vi "校准设置页.vi"() -> ()   [LabVIEW 2016, in "斯坦道总氮.lvlib"]
uses:
  <vilib>/Analysis/6fits.llb/Curve Fitting Criteria.ctl
  <vilib>/Analysis/NI_AALPro.lvlib
  <vilib>/ptbypt/NI_PtbyPt.lvlib
panel:
  out "校准状态显示":string caption="校准状态"
  out "刷新时间":string
  out "校准状态":T1(ring)
  out "模型刷新":bool
  in  "校准按钮":T2(radio)
  in  "校准导入":bool
  in  "辅助计算":bool
  in  "曲线模型":T3={"标液浓度1"=0.0, "测量吸光度1"=0.0, "样品1启用"=FALSE, "标液浓度2"=0.0, "测量吸光度2"=0.0, "样品2启用"=FALSE, "标液浓度3"=0.0, "测量吸光度3"=0.0, "样品3启用"=FALSE, "标液浓度4"=0.0, "测量吸光度4"=0.0, "样品4启用"=FALSE, "标液浓度5"=0.0, "测量吸光度5"=0.0, "样品5启用"=FALSE, "模型"=enum."线性", "精度"=4.0, "XY图"=[], "拟合公式"="", "r^2"=0.0, "标样一校准时间"=timestamp(0 s since 1904-01-01), "标样二校准时间"=timestamp(0 s since 1904-01-01), "标样三校准时间"=timestamp(0 s since 1904-01-01), "标样四校准时间"=timestamp(0 s since 1904-01-01), "标样五校准时间"=timestamp(0 s since 1904-01-01), "二次方程"={"c"=0.0, "x"=0.0, "x^2"=0.0}, "标定时间"=timestamp(0 s since 1904-01-01)} {"标定时间" format="%<%m/%d/%y %H:%M:%S>T"; "标样五校准时间" format="%<%m/%d/%y %H:%M:%S>T"; "标样四校准时间" format="%<%m/%d/%y %H:%M:%S>T"; "标样三校准时间" format="%<%m/%d/%y %H:%M:%S>T"; "标样二校准时间" format="%<%m/%d/%y %H:%M:%S>T"; "标样一校准时间" format="%<%m/%d/%y %H:%M:%S>T"; "r^2" format="%.7f"; "测量吸光度5" format="%#.6f"; "测量吸光度4" format="%#.6f"; "测量吸光度3" format="%#.6f"; "测量吸光度2" format="%#.6f"; "测量吸光度1" format="%#.6f"}
  in  "测量模式":T4(ring)
  in  "参数下拉列表":u16(ring)
  in  "量程下拉列表":enum16{"低量程", "高量程"}(ring)
  # "校准时间"
  # "标液浓度"
  # "吸光值"
  # "空白"
  # "标样一"
  # "标样二"
  # "零点"
  # "跨度"
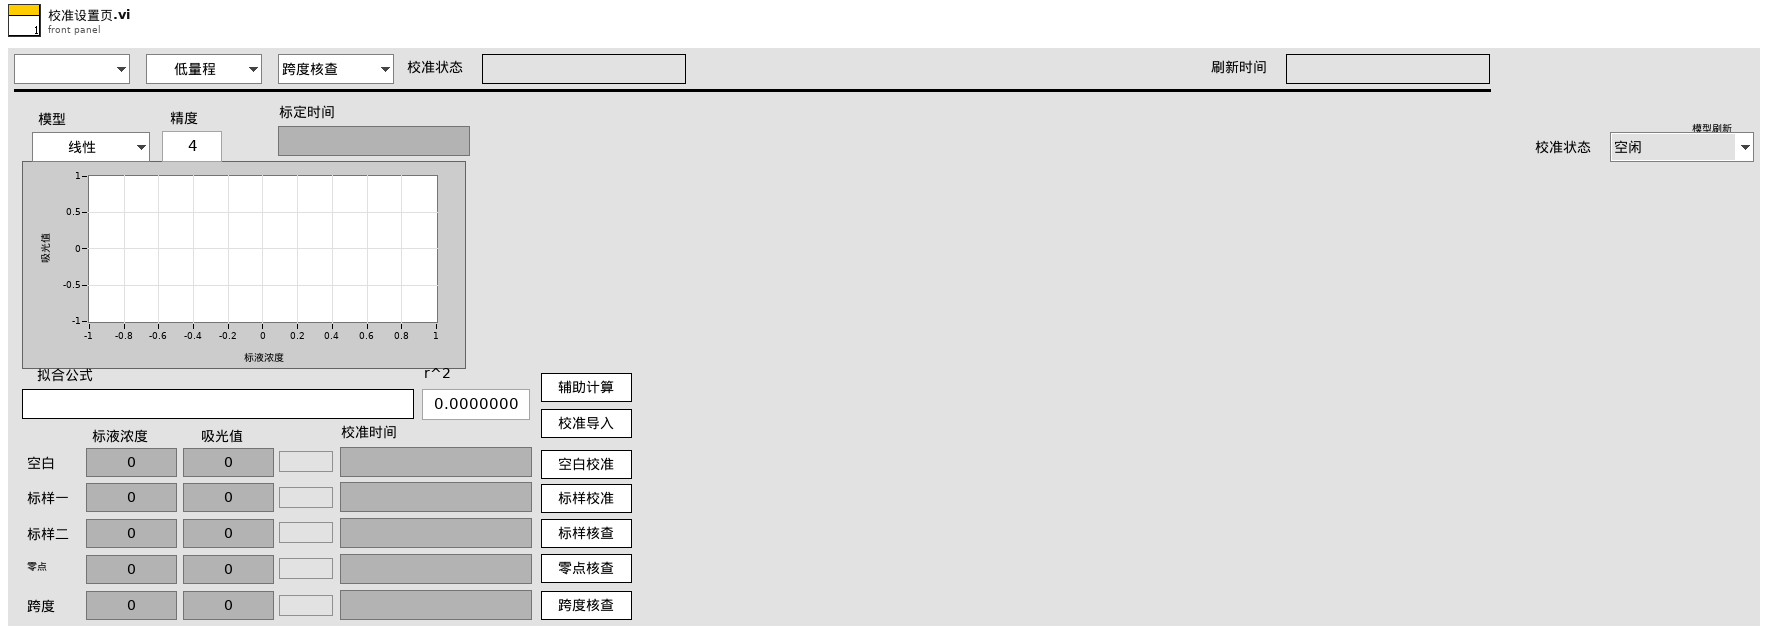
[diagram p1: front panel]
types:
  T1 = enum16{"空闲", "初始化", "校准启动", "校准运行中", "测试结束", "获取校准数据", "填充校准数据", "流程结束"}
  T2 = enum32{"未选择", "空白校准", "标样校准", "标样核查", "零点核查", "跨度核查"}
  T3 = cluster{"标液浓度1":dbl, "测量吸光度1":dbl, "样品1启用":bool, "标液浓度2":dbl, "测量吸光度2":dbl, "样品2启用":bool, "标液浓度3":dbl, "测量吸光度3":dbl, "样品3启用":bool, "标液浓度4":dbl, "测量吸光度4":dbl, "样品4启用":bool, "标液浓度5":dbl, "测量吸光度5":dbl, "样品5启用":bool, "模型":enum32{"线性", "多项式"}, "精度":dbl, "XY图":cluster{"X Values":dbl[], "Y Values":dbl[]}[], "拟合公式":string, "r^2":dbl, "标样一校准时间":timestamp, "标样二校准时间":timestamp, "标样三校准时间":timestamp, "标样四校准时间":timestamp, "标样五校准时间":timestamp, "二次方程":cluster{"c":dbl, "x":dbl, "x^2":dbl}, "标定时间":timestamp}
  T4 = enum16{"跨度核查", "水样测量", "零点核查", "标样核查", "加标回收", "快捷测试", "空白校准", "标样校准"}
  T5 = typedef "LVStringsAndValuesArrayTypeDef_U16.ctl" = cluster{"String":string, "Value":u16}[]
  T6 = enum8{"Enabled", "Disabled", "Disabled and Grayed Out"}
  T7 = cluster{"标液浓度1":dbl, "测量吸光度1":dbl, "样品1启用":bool, "标液浓度2":dbl, "测量吸光度2":dbl, "样品2启用":bool, "标液浓度3":dbl, "测量吸光度3":dbl, "样品3启用":bool, "标液浓度4":dbl, "测量吸光度4":dbl, "样品4启用":bool, "标液浓度5":dbl, "测量吸光度5":dbl, "样品5启用":bool, "模型":enum32{"线性", "多项式"}, "精度":dbl, "XY图":cluster{"X Values":dbl[], "Y Values":dbl[]}[], "拟合公式":string, "r^2":dbl, "标样一校准时间":timestamp, "标样二校准时间":timestamp, "标样三校准时间":timestamp, "标样四校准时间":timestamp, "标样五校准时间":timestamp, "二次方程":cluster{"c":dbl, "x":dbl, "x^2":dbl}, "标定时间":timestamp}[][]
  T8 = typedef "NI_AALPro.lvlib/Curve Fitting Criteria.ctl" = u16
  T9 = cluster{"标液浓度1":dbl, "测量吸光度1":dbl, "样品1启用":bool, "标液浓度2":dbl, "测量吸光度2":dbl, "样品2启用":bool, "标液浓度3":dbl, "测量吸光度3":dbl, "样品3启用":bool, "标液浓度4":dbl, "测量吸光度4":dbl, "样品4启用":bool, "标液浓度5":dbl, "测量吸光度5":dbl, "样品5启用":bool, "模型":enum32{"线性", "多项式"}, "精度":dbl, "XY图":cluster{"X Values":dbl[], "Y Values":dbl[]}[], "拟合公式":string, "r^2":dbl, "标样一校准时间":timestamp, "标样二校准时间":timestamp, "标样三校准时间":timestamp, "标样四校准时间":timestamp, "标样五校准时间":timestamp, "二次方程":cluster{"c":dbl, "x":dbl, "x^2":dbl}, "标定时间":timestamp}[]
  T10 = enum32{"Bad", "Idle", "Run top level", "Running"}
  T11 = cluster{"时间":timestamp, "标液值":dbl, "检测值":dbl, "吸光值":dbl}
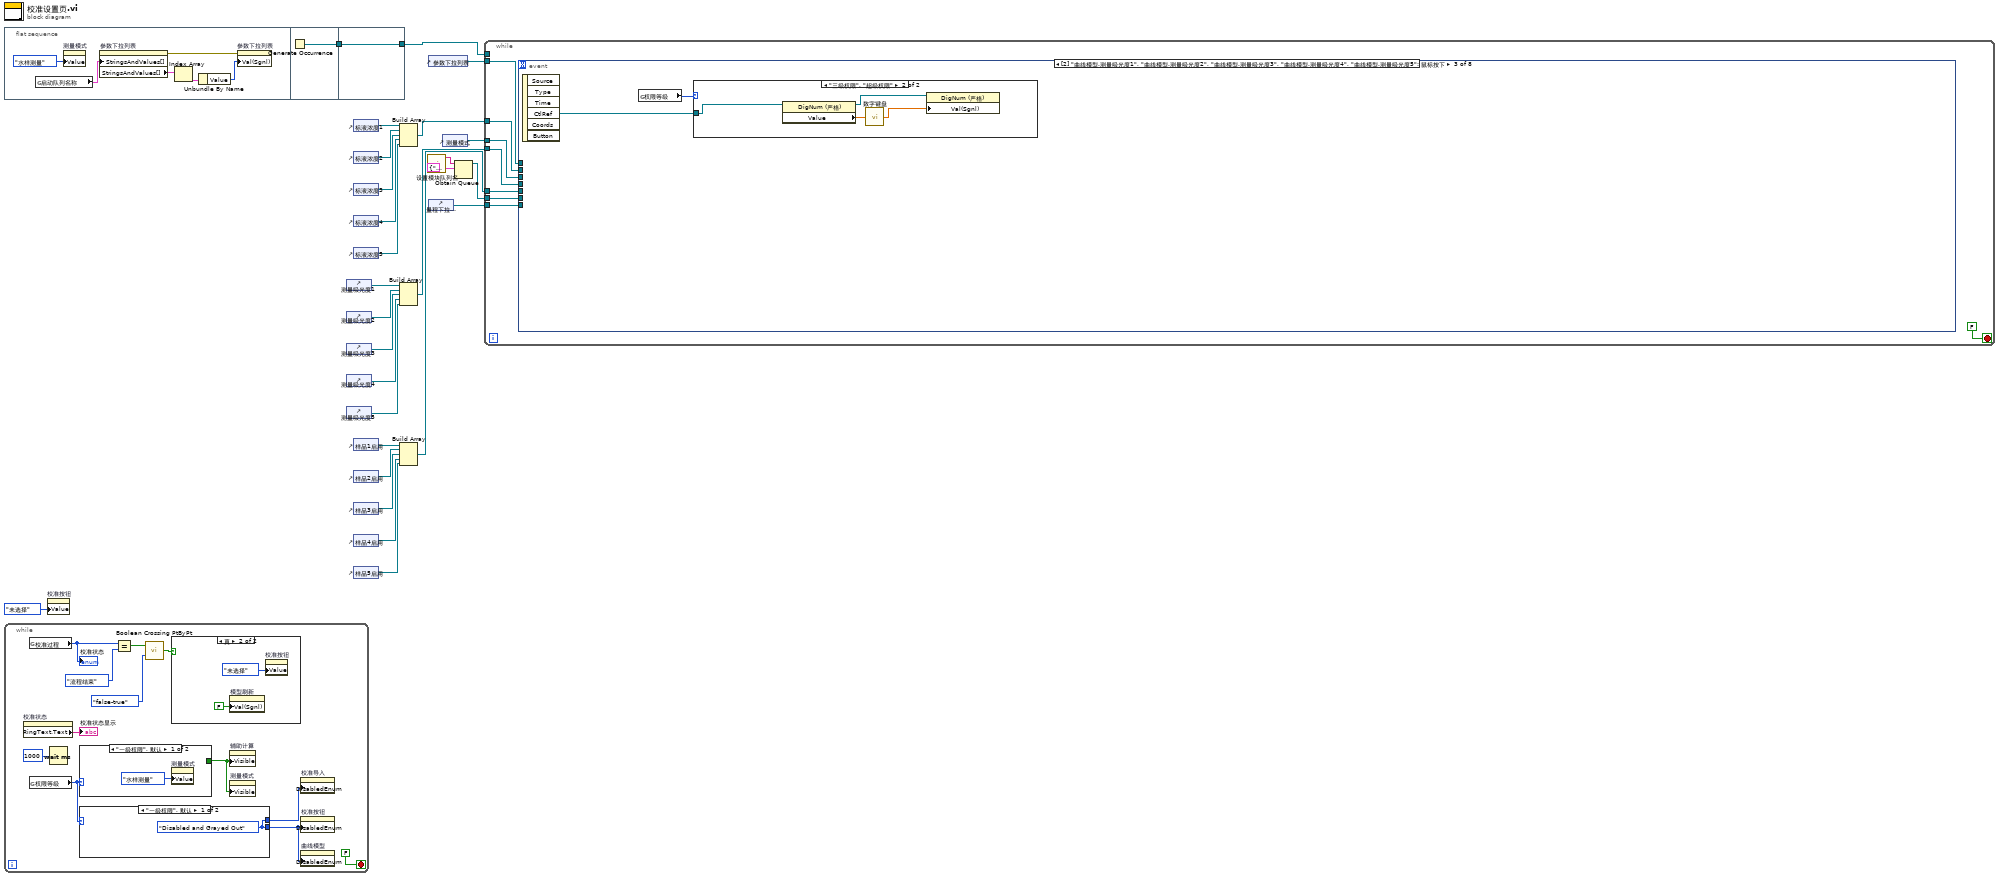
[diagram p0: block diagram]
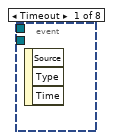
[diagram p2: hidden frame]
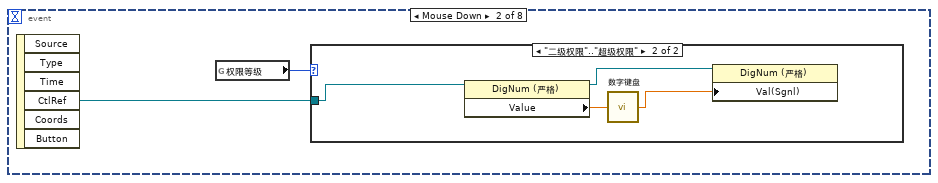
[diagram p3: hidden frame]
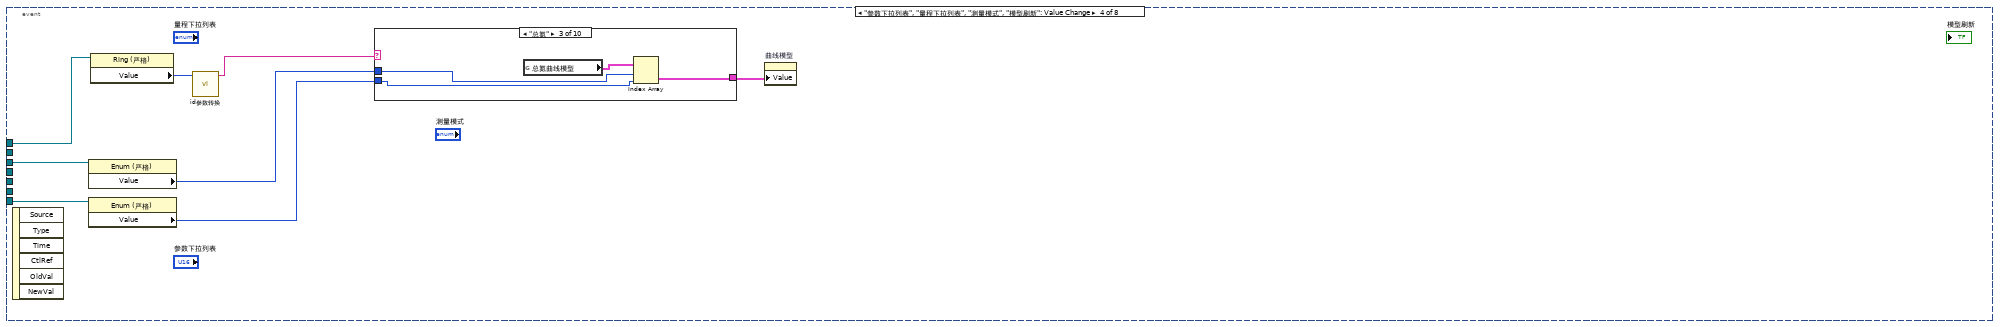
[diagram p6: hidden frame]
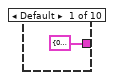
[diagram p7: hidden frame]
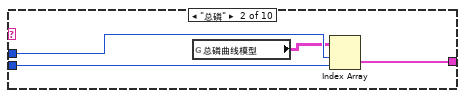
[diagram p8: hidden frame]
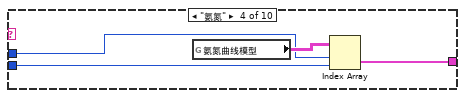
[diagram p9: hidden frame]
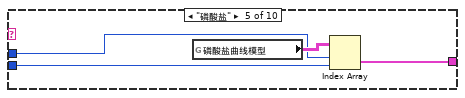
[diagram p10: hidden frame]
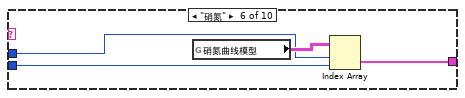
[diagram p11: hidden frame]
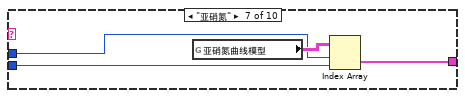
[diagram p12: hidden frame]
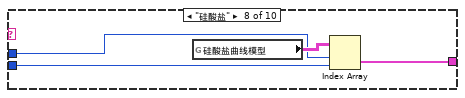
[diagram p13: hidden frame]
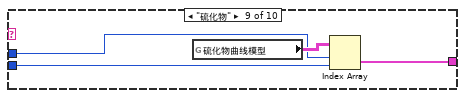
[diagram p14: hidden frame]
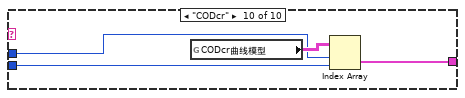
[diagram p15: hidden frame]
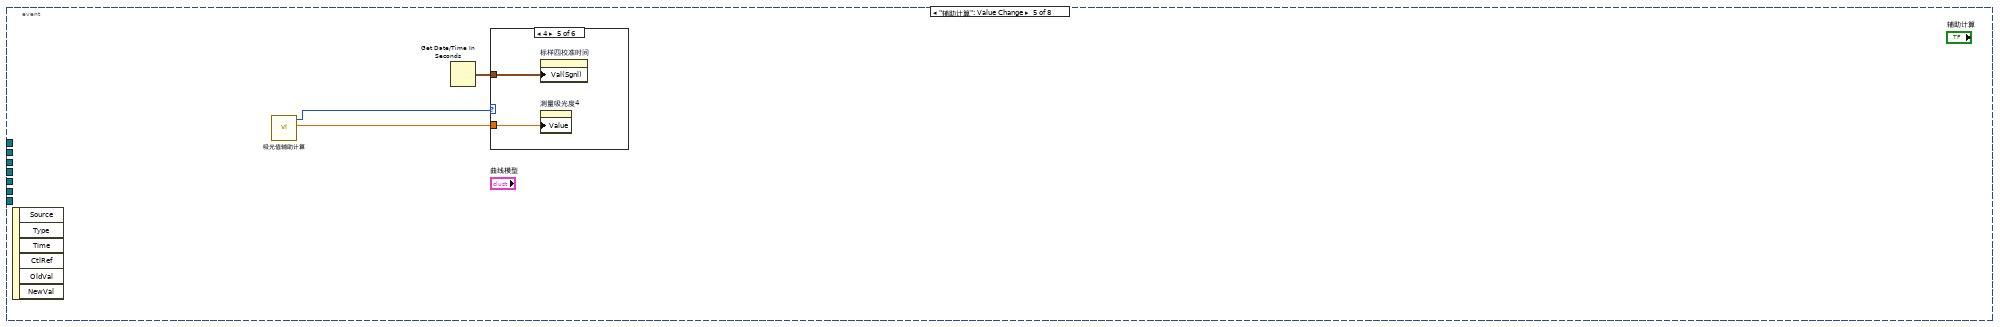
[diagram p16: hidden frame]
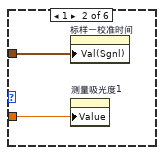
[diagram p18: hidden frame]
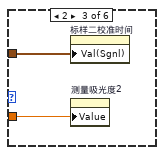
[diagram p19: hidden frame]
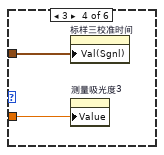
[diagram p20: hidden frame]
diagram:
  n1 = flat-sequence {
    tunnel: [w34] -> w27
    tunnel: [w35] -> w26
    tunnel: w27 -> [w35]
    frame #0 {
      n2 = global read "总磷总氮断电保存全局变量.vi" "启动队列名称"() -> (w29:cluster{"String":string, "Value":u16}[])
      n3 = property on="测量模式" class="Enum (严格)"("Value"=T4."水样测量" ("测量模式")) -> ()  [unwired: 2 in, 2 out]
      n4 = property on="参数下拉列表" class="Ring (严格)"("StringsAndValues[]"=w29) -> (error out=w32:errorcluster, "StringsAndValues[]"=w30:T5)  [unwired: 2 in, 1 out]
      n5 = Index Array(array=w30) -> (element=w31:cluster{"String":string, "Value":u16})  [unwired: 1 in]
      n6 = Unbundle By Name(w31) -> ("Value"=w33:u16)
      n7 = property on="参数下拉列表" class="Ring (严格)"(error in=w32, "Val(Sgnl)"=w33) -> ()  [unwired: 1 in, 2 out]
    }
    frame #1 {
      n8 = Generate Occurrence() -> (w34:refnum<k4>)
    }
    frame #2 {
    }
  }
  n9 = while {
    stop <- FALSE stop-if-true
    n10 = property on="校准状态" class="Enum (严格)"() -> ("RingText.Text"=→"校准状态显示":string)  [unwired: 2 in, 2 out]
    n11 = global read "VAR总磷总氮全局变量.vi" "校准过程"() -> (w38:T1)
    "校准状态" <- w38
    n12 = global read "VAR总磷总氮全局变量.vi" "权限等级"() -> (w44:enum16{"一级权限", "二级权限", "三级权限", "超级权限"})
    n13 = Wait (ms)(milliseconds to wait=u32 1000 ("等待时间（毫秒）")) -> ()  [unwired: 1 out]
    n14 = case shown="\"一级权限\", 默认" w44 {
      tunnel: [_ TRUE ("可见")] -> w43
      frame "一级权限", Default {
        n15 = property on="测量模式" class="Enum (严格)"("Value"=T4."水样测量" ("测量模式")) -> ()  [unwired: 2 in, 2 out]
      }
      frame "三级权限", "超级权限" {
      }
    }
    n16 = case shown="\"一级权限\", 默认" w44 {
      tunnel: [w52 w53] -> w42
      tunnel: [w52 w53] -> w45
      frame "一级权限", Default {
        w52 = T6."Disabled and Grayed Out" ("禁用")
      }
      frame "二级权限".."超级权限" {
        w53 = T6."Enabled" ("禁用")
      }
    }
    n17 = Equal?(x=w38, y=T1."流程结束" ("校准过程")) -> (x = y?=w41:bool)
    n18 = call <vilib>:"Boolean Crossing PtByPt.vi"("direction"=enum16{"either", "false-true", "true-false"}."false-true", "input"=w41) -> ("crossing"=w39:bool)  [unwired: 1 in]
    n19 = case shown="真" w39 {
      frame False {
      }
      frame True {
        n20 = property on="模型刷新" class="Bool (严格)"("Val(Sgnl)"=FALSE ("值(信号)")) -> ()  [unwired: 2 in, 2 out]
        n21 = property on="校准按钮" class="RadioBtnsControl (严格)"("Value"=T2."未选择" ("校准按钮")) -> ()  [unwired: 2 in, 2 out]
      }
    }
    n22 = property on="辅助计算" class="Bool"("Visible"=w43) -> ()  [unwired: 2 in, 2 out]
    n23 = property on="测量模式" class="Enum (严格)"("Visible"=w43) -> ()  [unwired: 2 in, 2 out]
    n24 = property on="校准导入" class="Bool"("DisabledEnum"=w45) -> ()  [unwired: 2 in, 2 out]
    n25 = property on="校准按钮" class="RadioBtnsControl (严格)"("DisabledEnum"=w42) -> ()  [unwired: 2 in, 2 out]
    n26 = property on="曲线模型" class="Clust (严格)"("DisabledEnum"=w42) -> ()  [unwired: 2 in, 2 out]
  }
  n27 = property on="校准按钮" class="RadioBtnsControl (严格)"("Value"=T2."未选择" ("校准按钮")) -> ()  [unwired: 2 in, 2 out]
  n28 = control-ref of="测量吸光度1"() -> (w15:refnum<vi>)
  n29 = control-ref of="测量吸光度2"() -> (w16:refnum<vi>)
  n30 = control-ref of="测量吸光度3"() -> (w17:refnum<vi>)
  n31 = control-ref of="测量吸光度4"() -> (w18:refnum<vi>)
  n32 = control-ref of="测量吸光度5"() -> (w19:refnum<vi>)
  n33 = control-ref of="标液浓度1"() -> (w13:refnum<vi>)
  n34 = control-ref of="标液浓度2"() -> (w12:refnum<vi>)
  n35 = control-ref of="标液浓度3"() -> (w11:refnum<vi>)
  n36 = control-ref of="标液浓度4"() -> (w10:refnum<vi>)
  n37 = control-ref of="标液浓度5"() -> (w9:refnum<vi>)
  n38 = control-ref of="样品1启用"() -> (w25:refnum<vi>)
  n39 = control-ref of="样品2启用"() -> (w24:refnum<vi>)
  n40 = control-ref of="样品3启用"() -> (w23:refnum<vi>)
  n41 = control-ref of="样品4启用"() -> (w22:refnum<vi>)
  n42 = control-ref of="样品5启用"() -> (w21:refnum<vi>)
  n43 = Build Array(w13, w12, w11, w10, w9) -> (w8:refnum<vi>[])
  n44 = Build Array(w15, w16, w17, w18, w19) -> (w14:refnum<vi>[])
  n45 = Build Array(w25, w24, w23, w22, w21) -> (w20:refnum<vi>[])
  n46 = call "设置模块队列名.vi"() -> ("Msg"=w6:string)  [unwired: 5 in]
  n47 = control-ref of="参数下拉列表"() -> (w3:refnum<vi>)
  n48 = control-ref of="量程下拉列表"() -> (w1:refnum<vi>)
  n49 = control-ref of="测量模式"() -> (w2:refnum<vi>)
  n50 = Obtain Queue(name (unnamed)=w6, element data type=cluster{"命令":string, "data":variant} {"命令"="", "data"=variant}) -> (queue out=w5:refnum<queue>)  [unwired: 3 in, 2 out]
  n51 = while {
    tunnel: w26 -> [_]
    tunnel: w3 -> [w60]
    tunnel: w20 -> [w59]
    tunnel: w14 -> [w58]
    tunnel: w8 -> [w57]
    tunnel: w2 -> [w56]
    tunnel: w1 -> [w55]
    tunnel: w5 -> [w54]
    stop <- FALSE stop-if-true
    n52 = event shown="[2] \"曲线模型.测量吸光度1\", \"曲线模型.测量吸光度2\", \"曲线模型.测量吸光度3\", \"曲线模型.测量吸光度4\", \"曲线模型.测量吸光度5\": 鼠标按下" {
      selector: _ -> [_ _ _ _ _ _ _ _]
      dyn-events: _ -> [_ _ _ _ _ _ _ _]
      timeout: _ -> [_ _ _ _ _ _ _ _]
      tunnel: w60 -> [_ _ _ w80 _ w144 w190 w272]
      tunnel: w59 -> [_ _ _ _ _ _ w194 _]
      tunnel: w58 -> [_ _ _ _ _ _ w193 _]
      tunnel: w57 -> [_ _ _ _ _ _ w192 _]
      tunnel: w56 -> [_ _ _ w78 _ w142 w188 w267]
      tunnel: w55 -> [_ _ _ w77 _ w140 w186 w271]
      tunnel: w54 -> [_ _ _ _ _ _ _ w273]
      event Timeout {
        n53 = event-data() -> ()  [unwired: 1 in, 3 out]
      }
      event "曲线模型.标液浓度1", "曲线模型.标液浓度2", "曲线模型.标液浓度3", "曲线模型.标液浓度4", "曲线模型.标液浓度5", "曲线模型.精度": Mouse Down {
        n54 = event-data() -> ("CtlRef"=w63:refnum<vi>)  [unwired: 1 in, 5 out]
        n55 = global read "VAR总磷总氮全局变量.vi" "权限等级"() -> (w62:enum16{"一级权限", "二级权限", "三级权限", "超级权限"})
        n56 = case shown="\"二级权限\"..\"超级权限\"" w62 {
          tunnel: w63 -> [_ w67]
          frame "一级权限", Default {
          }
          frame "二级权限".."超级权限" {
            n57 = property class="DigNum (严格)"(reference=w67) -> (reference out=w65:refnum<vi>, "Value"=w66:dbl)  [unwired: 1 in, 1 out]
            n58 = call "数字键盘.vi"("OldNumber"=w66) -> ("NewNumber"=w64:dbl)
            n59 = property class="DigNum (严格)"(reference=w65, "Val(Sgnl)"=w64) -> ()  [unwired: 1 in, 2 out]
          }
        }
      }
      event "曲线模型.测量吸光度1", "曲线模型.测量吸光度2", "曲线模型.测量吸光度3", "曲线模型.测量吸光度4", "曲线模型.测量吸光度5": Mouse Down {
        n60 = event-data() -> ("CtlRef"=w69:refnum<vi>)  [unwired: 1 in, 5 out]
        n61 = global read "VAR总磷总氮全局变量.vi" "权限等级"() -> (w68:enum16{"一级权限", "二级权限", "三级权限", "超级权限"})
        n62 = case shown="\"三级权限\", \"超级权限\"" w68 {
          tunnel: w69 -> [_ w73]
          frame "一级权限", Default {
          }
          frame "三级权限", "超级权限" {
            n63 = property class="DigNum (严格)"(reference=w73) -> (reference out=w71:refnum<vi>, "Value"=w72:dbl)  [unwired: 1 in, 1 out]
            n64 = call "数字键盘.vi"("OldNumber"=w72) -> ("NewNumber"=w70:dbl)
            n65 = property class="DigNum (严格)"(reference=w71, "Val(Sgnl)"=w70) -> ()  [unwired: 1 in, 2 out]
          }
        }
      }
      event "参数下拉列表", "量程下拉列表", "测量模式", "模型刷新": Value Change {
        n66 = event-data() -> ()  [unwired: 1 in, 6 out]
        n67 = property class="Enum (严格)"(reference=w78) -> ("Value"=w75:T4)  [unwired: 1 in, 2 out]
        n68 = property class="Enum (严格)"(reference=w77) -> ("Value"=w74:enum16{"低量程", "高量程"})  [unwired: 1 in, 2 out]
        n69 = property class="Ring (严格)"(reference=w80) -> ("Value"=w81:u16)  [unwired: 1 in, 2 out]
        n70 = call "id参数转换.vi"("id"=w81) -> ("table输出"=w79:string)  [unwired: 9 in, 1 out]
        n71 = case shown="\"总氮\"" w79 {
          tunnel: w74 -> [_ w85 w90 w92 w96 w100 w104 w108 w112 w116]
          tunnel: w75 -> [_ w86 w89 w93 w97 w101 w105 w109 w113 w117]
          tunnel: [T3 {"标液浓度1"=0.0, "测量吸光度1"=0.0, "样品1启用"=FALSE, "标液浓度2"=0.0, "测量吸光度2"=0.0, "样品2启用"=FALSE, "标液浓度3"=0.0, "测量吸光度3"=0.0, "样品3启用"=FALSE, "标液浓度4"=0.0, "测量吸光度4"=0.0, "样品4启用"=FALSE, "标液浓度5"=0.0, "测量吸光度5"=0.0, "样品5启用"=FALSE, "模型"=enum."线性", "精度"=0.0, "XY图"=[], "拟合公式"="", "r^2"=0.0, "标样一校准时间"=timestamp(0 s since 1904-01-01), "标样二校准时间"=timestamp(0 s since 1904-01-01), "标样三校准时间"=timestamp(0 s since 1904-01-01), "标样四校准时间"=timestamp(0 s since 1904-01-01), "标样五校准时间"=timestamp(0 s since 1904-01-01), "二次方程"={"c"=0.0, "x"=0.0, "x^2"=0.0}, "标定时间"=timestamp(0 s since 1904-01-01)} ("总磷曲线模型") w83 w87 w91 w95 w99 w103 w107 w111 w115] -> w76
          frame Default {
          }
          frame "总磷" {
            n72 = global read "校准数据全局变量.vi" "总磷曲线模型"() -> (w84:T7)
            n73 = Index Array(array=w84, index (row)=w86, index (col)=w85) -> (element=w83:T3)
          }
          frame "总氮" {
            n74 = global read "校准数据全局变量.vi" "总氮曲线模型"() -> (w88:T7)
            n75 = Index Array(array=w88, index (row)=w89, index (col)=w90) -> (element=w87:T3)
          }
          frame "氨氮" {
            n76 = global read "校准数据全局变量.vi" "氨氮曲线模型"() -> (w94:T7)
            n77 = Index Array(array=w94, index (row)=w93, index (col)=w92) -> (element=w91:T3)
          }
          frame "磷酸盐" {
            n78 = global read "校准数据全局变量.vi" "磷酸盐曲线模型"() -> (w98:T7)
            n79 = Index Array(array=w98, index (row)=w97, index (col)=w96) -> (element=w95:T3)
          }
          frame "硝氮" {
            n80 = global read "校准数据全局变量.vi" "硝氮曲线模型"() -> (w102:T7)
            n81 = Index Array(array=w102, index (row)=w101, index (col)=w100) -> (element=w99:T3)
          }
          frame "亚硝氮" {
            n82 = global read "校准数据全局变量.vi" "亚硝氮曲线模型"() -> (w106:T7)
            n83 = Index Array(array=w106, index (row)=w105, index (col)=w104) -> (element=w103:T3)
          }
          frame "硅酸盐" {
            n84 = global read "校准数据全局变量.vi" "硅酸盐曲线模型"() -> (w110:T7)
            n85 = Index Array(array=w110, index (row)=w109, index (col)=w108) -> (element=w107:T3)
          }
          frame "硫化物" {
            n86 = global read "校准数据全局变量.vi" "硫化物曲线模型"() -> (w114:T7)
            n87 = Index Array(array=w114, index (row)=w113, index (col)=w112) -> (element=w111:T3)
          }
          frame "CODcr" {
            n88 = global read "校准数据全局变量.vi" "CODcr曲线模型"() -> (w118:T7)
            n89 = Index Array(array=w118, index (row)=w117, index (col)=w116) -> (element=w115:T3)
          }
        }
        n90 = property on="曲线模型" class="Clust (严格)"("Value"=w76) -> ()  [unwired: 2 in, 2 out]
      }
      event "辅助计算": Value Change {
        n91 = event-data() -> ()  [unwired: 1 in, 6 out]
        n92 = call "吸光值辅助计算.vi"() -> ("X"=w120:dbl, "吸光值导出"=w121:u16)  [unwired: 10 in]
        n93 = Get Date/Time In Seconds() -> (seconds since 1Jan1904=w119:timestamp)
        n94 = case shown="4" w121 {
          tunnel: w120 -> [_ w123 w125 w127 w129 w131]
          tunnel: w119 -> [_ w122 w124 w126 w128 w130]
          frame 0, Default {
          }
          frame 1 {
            n95 = property on="标样一校准时间" class="AbsTime (严格)"("Val(Sgnl)"=w122) -> ()  [unwired: 2 in, 2 out]
            n96 = property on="测量吸光度1" class="DigNum (严格)"("Value"=w123) -> ()  [unwired: 2 in, 2 out]
          }
          frame 2 {
            n97 = property on="标样二校准时间" class="AbsTime (严格)"("Val(Sgnl)"=w124) -> ()  [unwired: 2 in, 2 out]
            n98 = property on="测量吸光度2" class="DigNum (严格)"("Value"=w125) -> ()  [unwired: 2 in, 2 out]
          }
          frame 3 {
            n99 = property on="标样三校准时间" class="AbsTime (严格)"("Val(Sgnl)"=w126) -> ()  [unwired: 2 in, 2 out]
            n100 = property on="测量吸光度3" class="DigNum (严格)"("Value"=w127) -> ()  [unwired: 2 in, 2 out]
          }
          frame 4 {
            n101 = property on="标样四校准时间" class="AbsTime (严格)"("Val(Sgnl)"=w128) -> ()  [unwired: 2 in, 2 out]
            n102 = property on="测量吸光度4" class="DigNum (严格)"("Value"=w129) -> ()  [unwired: 2 in, 2 out]
          }
          frame 5 {
            n103 = property on="标样五校准时间" class="AbsTime (严格)"("Val(Sgnl)"=w130) -> ()  [unwired: 2 in, 2 out]
            n104 = property on="测量吸光度5" class="DigNum (严格)"("Value"=w131) -> ()  [unwired: 2 in, 2 out]
          }
        }
      }
      event "校准导入": Value Change {
        n105 = event-data() -> ()  [unwired: 1 in, 6 out]
        n106 = property class="Enum (严格)"(reference=w142) -> ("Value"=w141:T4)  [unwired: 1 in, 2 out]
        n107 = property class="Enum (严格)"(reference=w140) -> ("Value"=w139:enum16{"低量程", "高量程"})  [unwired: 1 in, 2 out]
        n108 = property class="Ring (严格)"(reference=w144) -> ("Value"=w143:u16)  [unwired: 1 in, 2 out]
        n109 = property on="二次方程" class="Clust (严格)"() -> ("Value"=w133:cluster{"c":dbl, "x":dbl, "x^2":dbl})  [unwired: 2 in, 2 out]
        n110 = Unbundle By Name(w133) -> ("x^2"=w135:dbl, "x"=w136:dbl, "c"=w137:dbl)
        n111 = Bundle By Name(cluster=cluster{"X^2":dbl, "X":dbl, "b":dbl} {"X^2"=0.0, "X"=0.0, "b"=0.0} ("公式"), "X^2"=w135, "X"=w136, "b"=w137) -> (w132:cluster{"X^2":dbl, "X":dbl, "b":dbl})
        n112 = global read "VAR总磷总氮全局变量.vi" "权限等级"() -> (w138:enum16{"一级权限", "二级权限", "三级权限", "超级权限"})
        n113 = case shown="\"三级权限\", \"超级权限\"" w138 {
          tunnel: w143 -> [w153 w184]
          tunnel: w141 -> [w152 w183]
          tunnel: w139 -> [w151 w182]
          tunnel: w132 -> [w145 _]
          frame "一级权限", Default {
            n114 = Cluster To Array(cluster=w145) -> (array=w150:dbl[])
            n115 = Add Array Elements(numeric array=w150) -> (sum=w149:dbl)
            n116 = Equal To 0?(x=w149) -> (x = 0?=w147:bool)
            n117 = Not A Number/Path/Refnum?(number/path/refnum=w149) -> (NaN/Path/Refnum?=w148:bool)
            n118 = Or(x=w147, y=w148) -> (x .or. y?=w146:bool)
            n119 = case shown="假" w146 {
              tunnel: w153 -> [w159 _]
              tunnel: w152 -> [w158 _]
              tunnel: w151 -> [w157 _]
              tunnel: w145 -> [w154 _]
              frame False {
                n120 = Two Button Dialog(message="请再一次确认是否导入" ("消息")) -> (T button?=w155:bool)  [unwired: 2 in]
                n121 = case shown="真" w155 {
                  tunnel: w159 -> [_ w161]
                  tunnel: w158 -> [_ w167]
                  tunnel: w157 -> [_ w160]
                  tunnel: w154 -> [_ w162]
                  frame False {
                  }
                  frame True {
                    n122 = for {
                      N: 8 -> [_]
                      tunnel: w161 -> [w173]
                      tunnel: w167 -> [_]
                      tunnel: w160 -> [w172]
                      shift-right: [w171] -> w165
                      shift-left: errorcluster {"status"=FALSE, "code"=0, "source"=""} ("error out") -> [w168]
                      tunnel: w162 -> [w169]
                      i -> [w170]
                      n123 = call "总磷总氮公式写入.vi"("公式"=w169, "error in (no error)"=w168, "量程"=w172, "测量模式"=w170, "测量参数"=w173) -> ("error out"=w171:errorcluster)  [unwired: 6 in]
                    }
                    n124 = case shown="无错误" w165 {
                      tunnel: ["写入成功" "写入失败"] -> w166
                      tunnel: w161 -> [w177 _]
                      tunnel: w160 -> [w176 _]
                      frame No Error {
                        n125 = Get Date/Time In Seconds() -> (seconds since 1Jan1904=w178:timestamp)
                        n126 = property on="标定时间" class="AbsTime (严格)"("Val(Sgnl)"=w178) -> (error out=w174:errorcluster)  [unwired: 2 in, 1 out]
                        n127 = property on="曲线模型" class="Clust (严格)"(error in=w174) -> ("Value"=w175:T3)  [unwired: 1 in, 2 out]
                        n128 = call "校准记录.vi"("曲线模型"=w175, "量程"=w176, "校准参数"=w177) -> ()  [unwired: 8 in, 1 out]
                      }
                      frame Error {
                      }
                    }
                    n129 = One Button Dialog(message=w166) -> ()  [unwired: 1 in, 1 out]
                  }
                }
              }
              frame True {
                n130 = One Button Dialog(message="校准数据异常，请重新校准！" ("消息")) -> ()  [unwired: 1 in, 1 out]
              }
            }
          }
          frame "三级权限", "超级权限" {
            n131 = call "公式复合写入.vi"("量程下拉列表"=w182, "测量模式"=w183, "参数下拉列表"=w184) -> ()  [unwired: 9 in]
          }
        }
      }
      event "曲线模型": Value Change {
        n132 = event-data() -> ()  [unwired: 1 in, 6 out]
        n133 = flat-sequence {
          tunnel: w194 -> [w214]
          tunnel: w193 -> [w212]
          tunnel: w192 -> [w210]
          tunnel: [w197] -> w191
          tunnel: w190 -> [w197]
          tunnel: [w196] -> w189
          tunnel: w188 -> [w196]
          tunnel: [w195] -> w187
          tunnel: w186 -> [w195]
          tunnel: w191 -> [w230]
          tunnel: w189 -> [w227]
          tunnel: w187 -> [w226]
          frame #0 {
            w206 = T8 0 items=["最小二乘", "最小绝对残差", "Bisquare"] ("method")
            n134 = for {
              tunnel: w214 -> [w220] mode=indexing
              tunnel: [w219] -> w213 mode=indexing
              tunnel: w212 -> [w218] mode=indexing
              tunnel: [w217] -> w211 mode=indexing
              tunnel: w210 -> [w216] mode=indexing
              tunnel: [w215] -> w209 mode=indexing
              n135 = property class="DigNum (严格)"(reference=w216) -> ("Value"=w215:dbl)  [unwired: 1 in, 2 out]
              n136 = property class="DigNum (严格)"(reference=w218) -> ("Value"=w217:dbl)  [unwired: 1 in, 2 out]
              n137 = property class="Bool (严格)"(reference=w220) -> ("Value"=w219:bool)  [unwired: 1 in, 2 out]
            }
            n138 = property on="模型" class="Enum (严格)"() -> ("Value"=w208:enum32{"线性", "多项式"})  [unwired: 2 in, 2 out]
            n139 = property on="精度" class="DigNum (严格)"() -> ("Value"=w207:dbl)  [unwired: 2 in, 2 out]
            n140 = call "线性公式.vi"("精度"=w207, "模型"=w208, "method"=w206, "启用"=w213, "监测浓度"=w211, "标液浓度"=w209) -> ("Polynomial Coefficients 2"=w202:dbl[], "XY图"=w203:cluster{"X Values":dbl[], "Y Values":dbl[]}[], "r^2"=w204:dbl, "拟合方程"=w205:string)  [unwired: 2 in]
            n141 = property on="拟合公式" class="Str"("Value"=w205) -> ()  [unwired: 2 in, 2 out]
            n142 = property on="r^2" class="DigNum (严格)"("Value"=w204) -> ()  [unwired: 2 in, 2 out]
            n143 = property on="XY图" class="XYGraph (严格)"("Value"=w203) -> ()  [unwired: 2 in, 2 out]
            n144 = Index Array(array=w202) -> (element #1=w201:dbl, element #2=w200:dbl, element #3=w199:dbl)  [unwired: 3 in]
            n145 = Bundle("slope"=w201, "slope"=w200, "slope"=w199) -> (w198:cluster{"slope":dbl, "slope":dbl, "slope":dbl})  [unwired: 1 in]
            n146 = property on="二次方程" class="Clust (严格)"("Value"=w198) -> ()  [unwired: 2 in, 2 out]
          }
          frame #1 {
            n147 = property class="Enum (严格)"(reference=w227) -> ("Value"=w224:T4)  [unwired: 1 in, 2 out]
            n148 = property class="Enum (严格)"(reference=w226) -> ("Value"=w225:enum16{"低量程", "高量程"})  [unwired: 1 in, 2 out]
            n149 = property class="Ring (严格)"(reference=w230) -> ("Value"=w229:u16)  [unwired: 1 in, 2 out]
            n150 = property on="曲线模型" class="Clust (严格)"() -> ("Value"=w222:T3)  [unwired: 2 in, 2 out]
            n151 = call "id参数转换.vi"("id"=w229) -> ("table输出"=w228:string)  [unwired: 9 in, 1 out]
            n152 = Initialize Array(w222, 10 ("维数大小")) -> (w221:T9)
            n153 = case shown="\"总磷\"" w228 {
              tunnel: w221 -> [_ w231 w238 w240 w243 w247 w251 w255 w259 w264]
              tunnel: w225 -> [_ w234 w237 w241 w244 w248 w252 w256 w260 w265]
              tunnel: w224 -> [_ _ _ _ _ _ _ _ _ _]
              frame Default {
              }
              frame "总磷" {
                n154 = global read "校准数据全局变量.vi" "总磷曲线模型"() -> (w232:T7)
                n155 = Replace Array Subset(array=w232, new element=w231, index (col)=w234) -> (w233:T7)  [unwired: 1 in]
                n156 = global write "校准数据全局变量.vi" "总磷曲线模型"(w233) -> ()
              }
              frame "总氮" {
                n157 = global read "校准数据全局变量.vi" "总氮曲线模型"() -> (w236:T7)
                n158 = Replace Array Subset(array=w236, new element=w238, index (col)=w237) -> (w235:T7)  [unwired: 1 in]
                n159 = global write "校准数据全局变量.vi" "总氮曲线模型"(w235) -> ()
              }
              frame "氨氮" {
                n160 = global read "校准数据全局变量.vi" "氨氮曲线模型"() -> (w242:T7)
                n161 = Replace Array Subset(array=w242, new element=w240, index (col)=w241) -> (w239:T7)  [unwired: 1 in]
                n162 = global write "校准数据全局变量.vi" "氨氮曲线模型"(w239) -> ()
              }
              frame "磷酸盐" {
                n163 = global read "校准数据全局变量.vi" "磷酸盐曲线模型"() -> (w246:T7)
                n164 = Replace Array Subset(array=w246, new element=w243, index (col)=w244) -> (w245:T7)  [unwired: 1 in]
                n165 = global write "校准数据全局变量.vi" "磷酸盐曲线模型"(w245) -> ()
              }
              frame "硝氮" {
                n166 = global read "校准数据全局变量.vi" "硝氮曲线模型"() -> (w250:T7)
                n167 = Replace Array Subset(array=w250, new element=w247, index (col)=w248) -> (w249:T7)  [unwired: 1 in]
                n168 = global write "校准数据全局变量.vi" "硝氮曲线模型"(w249) -> ()
              }
              frame "亚硝氮" {
                n169 = global read "校准数据全局变量.vi" "亚硝氮曲线模型"() -> (w254:T7)
                n170 = Replace Array Subset(array=w254, new element=w251, index (col)=w252) -> (w253:T7)  [unwired: 1 in]
                n171 = global write "校准数据全局变量.vi" "亚硝氮曲线模型"(w253) -> ()
              }
              frame "硅酸盐" {
                n172 = global read "校准数据全局变量.vi" "硅酸盐曲线模型"() -> (w258:T7)
                n173 = Replace Array Subset(array=w258, new element=w255, index (col)=w256) -> (w257:T7)  [unwired: 1 in]
                n174 = global write "校准数据全局变量.vi" "硅酸盐曲线模型"(w257) -> ()
              }
              frame "硫化物" {
                n175 = global read "校准数据全局变量.vi" "硫化物曲线模型"() -> (w262:T7)
                n176 = Replace Array Subset(array=w262, new element=w259, index (col)=w260) -> (w261:T7)  [unwired: 1 in]
                n177 = global write "校准数据全局变量.vi" "硫化物曲线模型"(w261) -> ()
              }
              frame "CODcr" {
                n178 = global read "校准数据全局变量.vi" "CODcr曲线模型"() -> (w266:T7)
                n179 = Replace Array Subset(array=w266, new element=w264, index (col)=w265) -> (w263:T7)  [unwired: 1 in]
                n180 = global write "校准数据全局变量.vi" "CODcr曲线模型"(w263) -> ()
              }
            }
          }
          frame #2 {
            n181 = call "校准数据写入配置文件.vi"() -> ()  [unwired: 11 in, 1 out]
          }
        }
        n182 = Format Date/Time String() -> (date/time string=→"刷新时间":string)  [unwired: 3 in]
      }
      event "校准按钮": Value Change {
        n183 = event-data() -> ("NewVal"=w268:T2)  [unwired: 1 in, 5 out]
        n184 = Not Equal?(x=w268, y=T2."未选择") -> (x != y?=w269:bool)
        n185 = case shown="真" w269 {
          tunnel: w273 -> [_ _]
          tunnel: w272 -> [_ w279]
          tunnel: w271 -> [_ w278]
          tunnel: w268 -> [_ w276]
          tunnel: w267 -> [_ w277]
          frame False {
          }
          frame True {
            n186 = Two Button Dialog(message="是否获取历史数据作为校准点" ("消息")) -> (T button?=w275:bool)  [unwired: 2 in]
            n187 = case shown="真" w275 {
              tunnel: w279 -> [w285 w316]
              tunnel: w278 -> [w284 _]
              tunnel: w277 -> [w283 _]
              tunnel: w276 -> [w282 w315]
              frame False {
                n188 = Two Button Dialog(message="按确认立刻启动校准" ("消息")) -> (T button?=w280:bool)  [unwired: 2 in]
                n189 = case shown="真" w280 {
                  tunnel: w285 -> [_ w296]
                  tunnel: w284 -> [_ w295]
                  tunnel: w283 -> [_ w294]
                  tunnel: w282 -> [_ w290]
                  frame False {
                  }
                  frame True {
                    n190 = property class="Enum (严格)"(reference=w294) -> ("Value"=w288:T4)  [unwired: 1 in, 2 out]
                    n191 = property class="Enum (严格)"(reference=w295) -> ("Value"=w287:enum16{"低量程", "高量程"})  [unwired: 1 in, 2 out]
                    n192 = property class="Ring (严格)"(reference=w296) -> ("Value"=w289:u16)  [unwired: 1 in, 2 out]
                    n193 = vi-ref "校准流程.vi"() -> (w291:refnum<vi>)
                    n194 = local read "曲线模型"() -> (w286:T3)
                    n195 = property class="VI"(reference=w291) -> ("Name"=w292:string, "Exec.State"=w293:T10)  [unwired: 1 in, 2 out]
                    n196 = case shown="\"Bad\", 默认" w293 {
                      tunnel: w292 -> [_ w309]
                      tunnel: w290 -> [_ w302]
                      tunnel: w289 -> [_ w301]
                      tunnel: w288 -> [_ w300]
                      tunnel: w287 -> [_ w299]
                      tunnel: w286 -> [_ w298]
                      frame "Bad", Default {
                        n197 = One Button Dialog(message="正在校准，请在校准完成后操作！" ("消息")) -> ()  [unwired: 1 in, 1 out]
                      }
                      frame "Idle" {
                        n198 = Open VI Reference(type specifier VI Refnum (for type only)=refnum<vi> refnum, vi path=w309, options=128 ("选项")) -> (vi reference=w307:refnum<vi>, error out=w306:errorcluster)  [unwired: 3 in]
                        n199 = call-by-ref "开始异步调用"(reference=w307, error in=w306, "校准模式"=w302, "参数下拉列表"=w301, "测量模式"=w300, "量程下拉列表"=w299, "曲线模型"=w298) -> (reference out=w304:refnum<vi>, error out=w305:errorcluster)  [unwired: 11 in]
                        n200 = Close Reference(reference=w304, error in (no error)=w305) -> ()  [unwired: 1 out]
                      }
                    }
                  }
                }
              }
              frame True {
                n201 = case shown="\"跨度核查\"" w315 {
                  tunnel: [T4."水样测量" ("测量模式") T4."空白校准" ("测量模式") T4."标样校准" ("测量模式") T4."标样核查" ("测量模式") T4."零点核查" ("测量模式") T4."跨度核查" ("测量模式")] -> w312
                  frame "未选择", Default {
                  }
                  frame "空白校准" {
                  }
                  frame "标样校准" {
                  }
                  frame "标样核查" {
                  }
                  frame "零点核查" {
                  }
                  frame "跨度核查" {
                  }
                }
                n202 = property class="Ring (严格)"(reference=w316) -> ("Value"=w314:u16)  [unwired: 1 in, 2 out]
                n203 = call "id参数转换.vi"("id"=w314) -> ("table输出"=w313:string)  [unwired: 9 in, 1 out]
                n204 = call "校准数据选择表.vi"("测量模式"=w312, "table"=w313) -> ("布尔"=w311:bool, "输出"=w310:T11)  [unwired: 8 in]
                n205 = case shown="真" w311 {
                  tunnel: w310 -> [_ w320]
                  tunnel: w315 -> [_ w323]
                  frame False {
                  }
                  frame True {
                    n206 = Unbundle By Name(w320) -> ("时间"=w319:timestamp, "标液值"=w318:dbl, "吸光值"=w317:dbl)
                    n207 = property on="曲线模型" class="Clust (严格)"() -> ("Value"=w321:T3)  [unwired: 2 in, 2 out]
                    n208 = case shown="\"标样核查\"" w323 {
                      tunnel: [w324 w328 w333 w338 w343 w348] -> w322
                      tunnel: w321 -> [w324 w329 w334 w339 w344 w349]
                      tunnel: w319 -> [_ w327 w332 w337 w342 w347]
                      tunnel: w318 -> [_ w326 w331 w336 w341 w346]
                      tunnel: w317 -> [_ w325 w330 w335 w340 w345]
                      frame "未选择", Default {
                      }
                      frame "空白校准" {
                        n209 = Bundle By Name(cluster=w329, "标样一校准时间"=w327, "标液浓度1"=w326, "测量吸光度1"=w325) -> (w328:T3)
                      }
                      frame "标样校准" {
                        n210 = Bundle By Name(cluster=w334, "标样二校准时间"=w332, "标液浓度2"=w331, "测量吸光度2"=w330) -> (w333:T3)
                      }
                      frame "标样核查" {
                        n211 = Bundle By Name(cluster=w339, "标样三校准时间"=w337, "标液浓度3"=w336, "测量吸光度3"=w335) -> (w338:T3)
                      }
                      frame "零点核查" {
                        n212 = Bundle By Name(cluster=w344, "标样四校准时间"=w342, "标液浓度4"=w341, "测量吸光度4"=w340) -> (w343:T3)
                      }
                      frame "跨度核查" {
                        n213 = Bundle By Name(cluster=w349, "标样五校准时间"=w347, "标液浓度5"=w346, "测量吸光度5"=w345) -> (w348:T3)
                      }
                    }
                    n214 = property on="曲线模型" class="Clust (严格)"("Val(Sgnl)"=w322) -> ()  [unwired: 2 in, 2 out]
                  }
                }
              }
            }
          }
        }
      }
    }
  }
